vi "Flush.vi"(6 "returnNodes":bool, 8 "error in (no error)":errorcluster, 11 "Tree in":refnum<class "Tree.lvclass">) -> (0 "error out":errorcluster, 2 "Nodes":refnum<data-value>[](array[refnum]), 3 "Tree out":refnum<class "Tree.lvclass">)   [LabVIEW 2013, in "Tree.lvclass"]
uses:
  Tree.lvclass
  LLNode/LLNode.lvclass
  Tree.lvclass/Tree.ctl
  SearchMethod.ctl
  TreeNode/TreeNode.lvclass
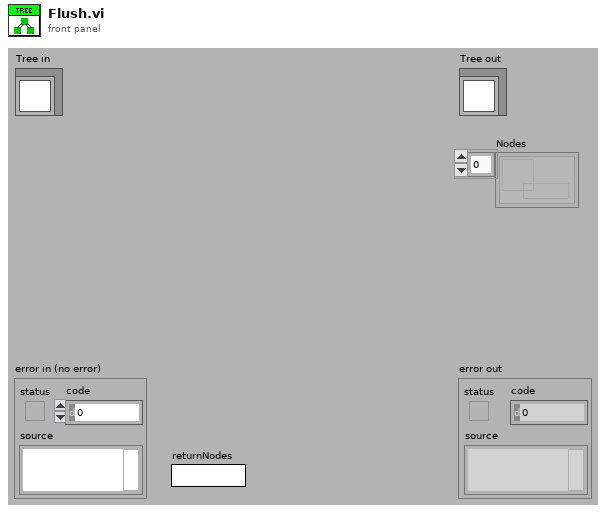
[diagram p1: front panel]
types:
  T1 = typedef "Tree.lvclass/SearchMethod.ctl" = enum16{"Breadth (First)", "Depth (First)", "Best First", "Breadth (Exhaustive)", "Depth (Exhaustive)"}
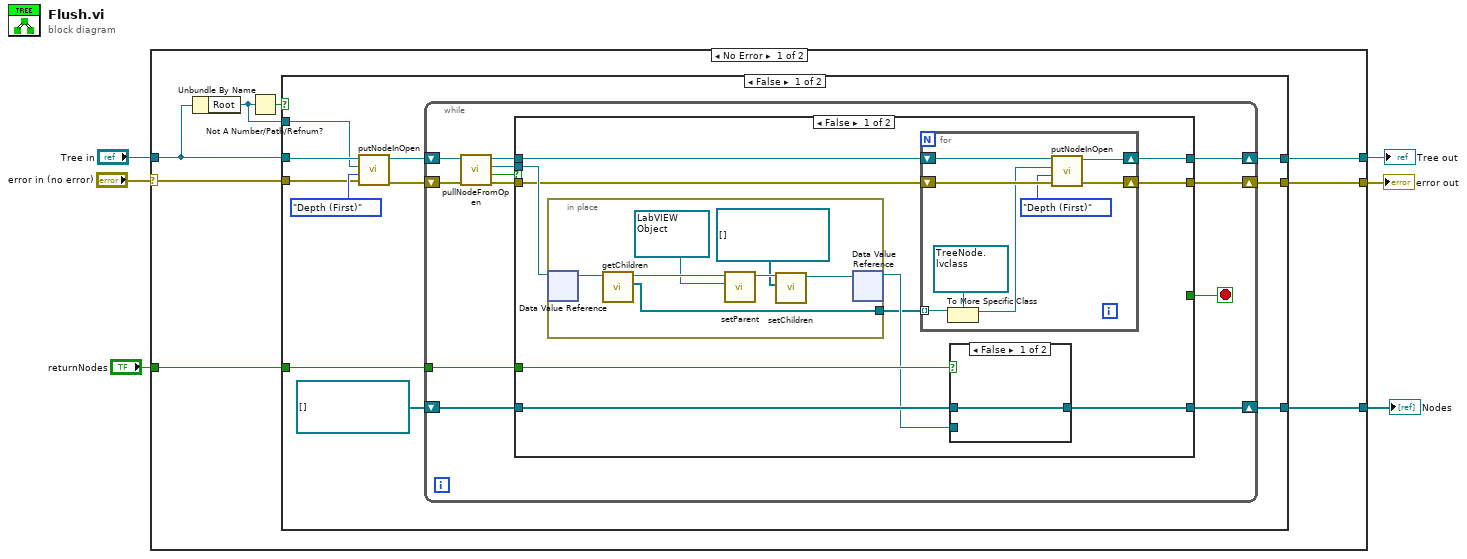
[diagram p0: block diagram]
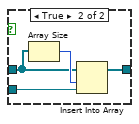
[diagram p2: hidden frame]
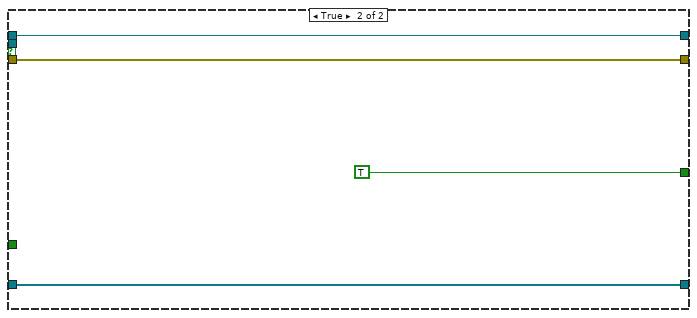
[diagram p3: hidden frame]
diagram:
  n1 = case shown="No Error" "error in (no error)" {
    selector: "error in (no error)" -> [w11 w75]
    tunnel: [w7 w75] -> w5
    tunnel: [w9 w74] -> w3
    tunnel: "Tree in" -> [w13 w74]
    tunnel: "returnNodes" -> [w10 _]
    tunnel: [w8 _] -> w1
    frame No Error {
      n2 = Unbundle By Name(w13) -> ("Root"=w12:refnum<data-value>)
      n3 = Not A Number/Path/Refnum?(number/path/refnum=w12) -> (NaN/Path/Refnum?=w14:bool)
      n4 = case shown="False" w14 {
        tunnel: w13 -> [w25 w73]
        tunnel: w12 -> [w24 _]
        tunnel: w11 -> [w22 w72]
        tunnel: w10 -> [w18 _]
        tunnel: [w17 _] -> w8
        tunnel: [w16 w73] -> w9
        tunnel: [w15 w72] -> w7
        frame False {
          n5 = call "putNodeInOpen.vi"("error in (no error)"=w22, "SearchMethod"=SearchMethod."Depth (First)", "TreeNode"=w24, "Tree in"=w25) -> ("error out"=w20:errorcluster, "Tree out"=w21:refnum<class "Tree.lvclass">)  [unwired: 6 in]
          n6 = while {
            shift-right: [w33] -> w16
            shift-left: w21 -> [w37]
            shift-right: [w31] -> w15
            shift-left: w20 -> [w36]
            shift-right: [w28] -> w17
            shift-left: refnum<data-value>[] [] -> [w29]
            tunnel: w18 -> [w26]
            stop <- w27 stop-if-true
            n7 = call "pullNodeFromOpen.vi"("error in (no error)"=w36, "Tree in"=w37) -> ("error out"=w32:errorcluster, "empty"=w35:bool, "RemovedNode"=w30:refnum<data-value>, "Tree out"=w34:refnum<class "Tree.lvclass">)  [unwired: 6 in]
            n8 = case shown="False" w35 {
              tunnel: w34 -> [w41 w71]
              tunnel: [w39 w71] -> w33
              tunnel: w32 -> [w40 w70]
              tunnel: [w38 w70] -> w31
              tunnel: w30 -> [w47 _]
              tunnel: w29 -> [w45 w69]
              tunnel: [w44 w69] -> w28
              tunnel: [_ TRUE] -> w27
              tunnel: w26 -> [w46 _]
              frame False {
                n9 = in-place {
                  in-place-border: [w61] -> w42
                  n10 = in-place-dvr #1(w47) -> (w67:refnum<class "TreeNode.lvclass">)  [unwired: 1 out]
                  n11 = call "getChildren.vi"("TreeNode in"=w67) -> ("Children"=w61:refnum<data-value>[], "TreeNode out"=w66:refnum<class "TreeNode.lvclass">)  [unwired: 8 in, 1 out]
                  n12 = call "setParent.vi"("Parent"=refnum<data-value> refnum, "TreeNode in"=w66) -> ("TreeNode out"=w65:refnum<class "TreeNode.lvclass">)  [unwired: 8 in, 1 out]
                  n13 = call "setChildren.vi"("Children"=refnum<data-value>[] [], "TreeNode in"=w65) -> ("TreeNode out"=w62:refnum<class "TreeNode.lvclass">)  [unwired: 8 in, 1 out]
                  n14 = in-place-dvr #1(w62) -> (w43:refnum<data-value>)  [unwired: 1 out]
                }
                n15 = for {
                  tunnel: w42 -> [w55] mode=indexing
                  shift-right: [w52] -> w39
                  shift-left: w41 -> [w53]
                  shift-right: [w50] -> w38
                  shift-left: w40 -> [w51]
                  n16 = To More Specific Class(target class=refnum<data-value> refnum ("RemovedNode"), reference=w55) -> (specific class reference=w49:refnum<data-value>)  [unwired: 1 in, 1 out]
                  n17 = call "putNodeInOpen.vi"("error in (no error)"=w51, "SearchMethod"=SearchMethod."Depth (First)", "TreeNode"=w49, "Tree in"=w53) -> ("error out"=w50:errorcluster, "Tree out"=w52:refnum<class "Tree.lvclass">)  [unwired: 6 in]
                }
                n18 = case shown="False" w46 {
                  tunnel: w45 -> [w56 w58]
                  tunnel: [w56 w60] -> w44
                  tunnel: w43 -> [_ w57]
                  frame False {
                  }
                  frame True {
                    n19 = Array Size(array=w58) -> (size(s)=w59:i32)
                    n20 = Insert Into Array(array=w58, index=w59, new element=w57) -> (w60:refnum<data-value>[])
                  }
                }
              }
              frame True {
              }
            }
          }
        }
        frame True {
        }
      }
    }
    frame Error {
    }
  }
  "error out" <- w5
  "Tree out" <- w3
  "Nodes" <- w1
